vi "Autoscore.vi"   [LabVIEW 2018]
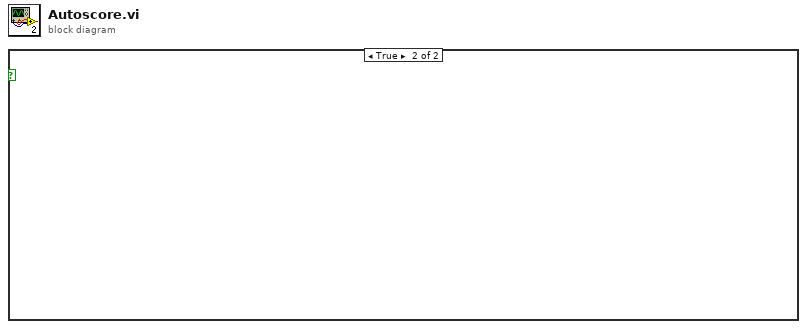
[diagram p0: block diagram]
diagram:
  n1 = case shown="True" {
    selector: _ -> [_ _]
    frame False {
    }
    frame True {
    }
  }
